vi "Get LVClass Path.vi"(11 "Manifestation Writer in":refnum<class "Manifestation Writer.lvclass">) -> (2 "LVClass Path":path, 3 "Manifestation Writer out":refnum<class "Manifestation Writer.lvclass">)   [LabVIEW 2013, in "Manifestation Writer.lvclass"]
uses:
  Manifestation Writer.lvclass
  Manifestation Writer.lvclass/Manifestation Writer.ctl
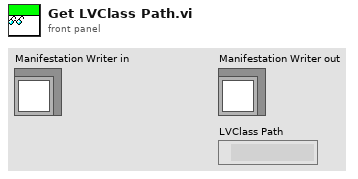
[diagram p1: front panel]
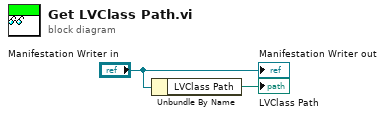
[diagram p0: block diagram]
diagram:
  n1 = Unbundle By Name("Manifestation Writer in") -> ("LVClass Path"=→"LVClass Path":path)
  "Manifestation Writer out" <- "Manifestation Writer in"
